vi "1.1 Act Debug Updater Loop.vi"   [LabVIEW 2011]
uses:
  2-Low Neurons/2.1 Act Debug.ctl
  1.0-Hindbrain Global.vi
types:
  T1 = typedef "2.1 Act Debug.ctl" = cluster{"Drive":cluster{"2.1 Drive Control Voltage":fxp<+/-,20,5>, "2.1 Drive PID Output":fxp<+/-,20,5>, "2.1.1 Drive Error":fxp<+/-,18,1>, "2.1.1 Drive Error I":fxp<+/-,64,46>, "2.1.1 Drive Error D":fxp<+/-,18,1>, "Motor Speed Integer":fxp<+/-,10,8>, "Drive Position Integer":i32}, "Steering":cluster{"2.1  Steering Control Voltage":fxp<+/-,20,5>, "2.1  Steering Lead Output":fxp<+/-,20,5>, "Steering V":fxp<+/-,10,8>, "Steering Position Integer":i32, "2.1.2 sqrt(10)s+bdt":fxp<+/-,18,20>, "2.1.2 (sqrt(10)s+bdt)/(s/sqrt(10)+bdt)":fxp<+/-,20,22>, "2.1.2 s(sqrt(10)s+bdt)/(s/sqrt(10)+bdt)":fxp<+/-,20,22>}, "Lidar":cluster{"2.1  Lidar Control Voltage":fxp<+/-,20,5>, "2.1  Lidar PID Output":fxp<+/-,20,5>, "2.1.3 Lidar Error":fxp<+/-,18,1>, "2.1.3 Lidar Error I":fxp<+/-,64,46>, "2.1.3 Lidar Error D":fxp<+/-,18,1>, "Lidar Position Integer":i32, "Lidar Motor Position Integer":i32}}
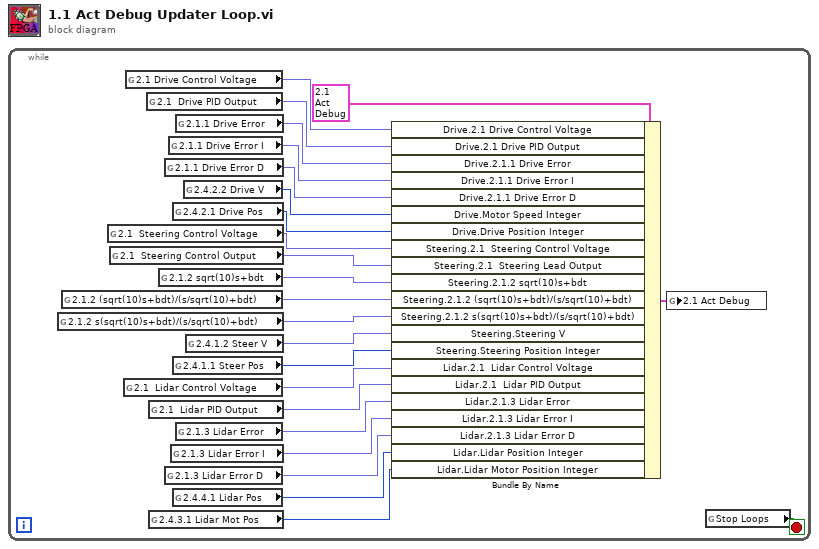
[diagram p0: block diagram]
diagram:
  n1 = while {
    stop <- w5 stop-if-true
    n2 = global read "1.0-Hindbrain Global.vi" "2.1.2 s(sqrt(10)s+bdt)/(s/sqrt(10)+bdt)"() -> (w3:fxp<+/-,20,22>)
    n3 = global read "1.0-Hindbrain Global.vi" "2.1.2 (sqrt(10)s+bdt)/(s/sqrt(10)+bdt)"() -> (w2:fxp<+/-,20,22>)
    n4 = global read "1.0-Hindbrain Global.vi" "2.1  Steering Control Voltage"() -> (w15:fxp<+/-,20,5>)
    n5 = global read "1.0-Hindbrain Global.vi" "2.1  Steering Control Output"() -> (w1:fxp<+/-,20,5>)
    n6 = global read "1.0-Hindbrain Global.vi" "2.1  Lidar Control Voltage"() -> (w6:fxp<+/-,20,5>)
    n7 = global read "1.0-Hindbrain Global.vi" "2.1 Drive Control Voltage"() -> (w22:fxp<+/-,20,5>)
    n8 = global read "1.0-Hindbrain Global.vi" "2.1  Drive PID Output"() -> (w21:fxp<+/-,20,5>)
    n9 = global read "1.0-Hindbrain Global.vi" "2.1  Lidar PID Output"() -> (w10:fxp<+/-,20,5>)
    n10 = global read "1.0-Hindbrain Global.vi" "2.4.3.1 Lidar Mot Pos"() -> (w7:i32)
    n11 = global read "1.0-Hindbrain Global.vi" "2.1.2 sqrt(10)s+bdt"() -> (w4:fxp<+/-,18,20>)
    n12 = global read "1.0-Hindbrain Global.vi" "2.1.1 Drive Error D"() -> (w18:fxp<+/-,18,1>)
    n13 = global read "1.0-Hindbrain Global.vi" "2.1.3 Lidar Error D"() -> (w12:fxp<+/-,18,1>)
    n14 = global read "1.0-Hindbrain Global.vi" "2.1.1 Drive Error I"() -> (w19:fxp<+/-,64,46>)
    n15 = global read "1.0-Hindbrain Global.vi" "2.1.3 Lidar Error I"() -> (w13:fxp<+/-,64,46>)
    n16 = global read "1.0-Hindbrain Global.vi" "2.4.2.1 Drive Pos"() -> (w16:i64)
    n17 = global read "1.0-Hindbrain Global.vi" "2.4.1.1 Steer Pos"() -> (w8:i32)
    n18 = global read "1.0-Hindbrain Global.vi" "2.4.4.1 Lidar Pos"() -> (w9:i32)
    n19 = global read "1.0-Hindbrain Global.vi" "2.1.1 Drive Error"() -> (w20:fxp<+/-,18,1>)
    n20 = global read "1.0-Hindbrain Global.vi" "2.1.3 Lidar Error"() -> (w14:fxp<+/-,18,1>)
    n21 = global read "1.0-Hindbrain Global.vi" "2.4.2.2 Drive V"() -> (w17:i32)
    n22 = global read "1.0-Hindbrain Global.vi" "2.4.1.2 Steer V"() -> (w11:fxp<+/-,10,8>)
    n23 = Bundle By Name(cluster=T1 {"Drive"={"2.1 Drive Control Voltage"=0.0, "2.1 Drive PID Output"=0.0, "2.1.1 Drive Error"=0.0, "2.1.1 Drive Error I"=0.0, "2.1.1 Drive Error D"=0.0, "Motor Speed Integer"=0.0, "Drive Position Integer"=0}, "Steering"={"2.1  Steering Control Voltage"=0.0, "2.1  Steering Lead Output"=0.0, "Steering V"=0.0, "Steering Position Integer"=0, "2.1.2 sqrt(10)s+bdt"=0.0, "2.1.2 (sqrt(10)s+bdt)/(s/sqrt(10)+bdt)"=0.0, "2.1.2 s(sqrt(10)s+bdt)/(s/sqrt(10)+bdt)"=0.0}, "Lidar"={"2.1  Lidar Control Voltage"=0.0, "2.1  Lidar PID Output"=0.0, "2.1.3 Lidar Error"=0.0, "2.1.3 Lidar Error I"=0.0, "2.1.3 Lidar Error D"=0.0, "Lidar Position Integer"=0, "Lidar Motor Position Integer"=0}} ("2.1 Act Debug"), "Drive.2.1 Drive Control Voltage"=w22, "Drive.2.1 Drive PID Output"=w21, "Drive.2.1.1 Drive Error"=w20, "Drive.2.1.1 Drive Error I"=w19, "Drive.2.1.1 Drive Error D"=w18, "Drive.Motor Speed Integer"=w17, "Drive.Drive Position Integer"=w16, "Steering.2.1  Steering Control Voltage"=w15, "Steering.2.1  Steering Lead Output"=w1, "Steering.2.1.2 sqrt(10)s+bdt"=w4, "Steering.2.1.2 (sqrt(10)s+bdt)/(s/sqrt(10)+bdt)"=w2, "Steering.2.1.2 s(sqrt(10)s+bdt)/(s/sqrt(10)+bdt)"=w3, "Steering.Steering V"=w11, "Steering.Steering Position Integer"=w8, "Lidar.2.1  Lidar Control Voltage"=w6, "Lidar.2.1  Lidar PID Output"=w10, "Lidar.2.1.3 Lidar Error"=w14, "Lidar.2.1.3 Lidar Error I"=w13, "Lidar.2.1.3 Lidar Error D"=w12, "Lidar.Lidar Position Integer"=w9, "Lidar.Lidar Motor Position Integer"=w7) -> (w23:T1)
    n24 = global write "1.0-Hindbrain Global.vi" "2.1 Act Debug"(w23) -> ()
    n25 = global read "1.0-Hindbrain Global.vi" "Stop Loops"() -> (w5:bool)
  }
